vi "Divideby2.vi"(1 "Input":i16) -> (0 "Output":i16)   [LabVIEW 2017]
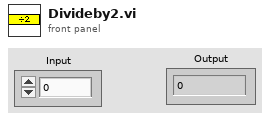
[diagram p1: front panel]
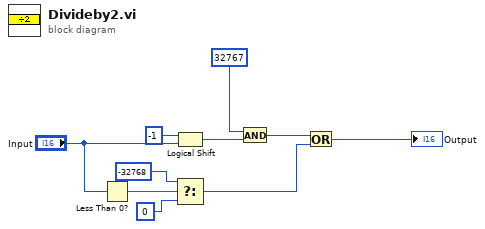
[diagram p0: block diagram]
diagram:
  n1 = Less Than 0?(x="Input") -> (x < 0?=w9:bool)
  n2 = Logical Shift(y=i16 -1, x="Input") -> (x << y=w2:i16)
  n3 = Select(t=i16 -32768 ("y"), s=w9, f=i16 0 ("y")) -> (s? t:f=w4:i16)
  n4 = And(x=i16 32767 ("y"), y=w2) -> (x .and. y?=w1:i16)
  n5 = Or(x=w1, y=w4) -> (x .or. y?=→"Output":i16)
